vi "DAQ simulation.vi"(5 "Sampling rate":dbl=18000.0, 7 "Samples per channel":i32=500, 8 "Delay time (Pulse width) ms":i32=10, 9 "index (row)":i32, 11 "Input data":dbl[][](array[numeric])) -> (1 "Stop":bool, 3 "Output":dbl[](array[numeric]))   [LabVIEW 2018]
panel:
  out "Waveform Graph":dbl[](graph)
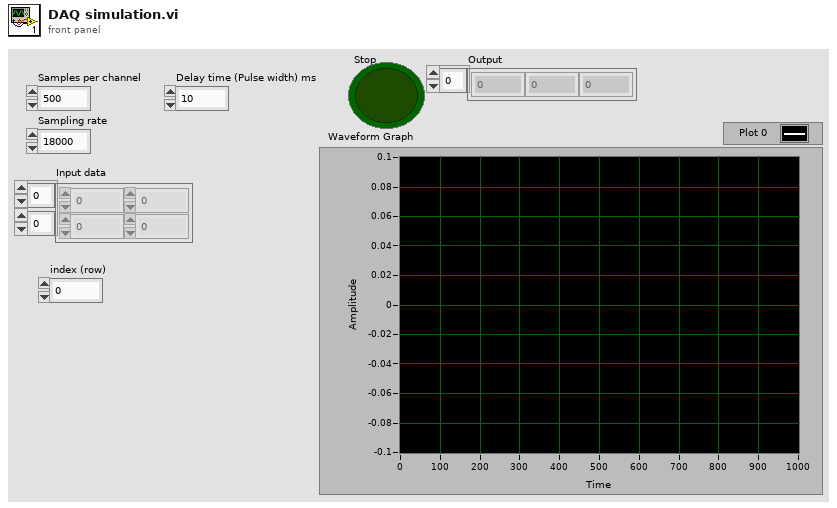
[diagram p1: front panel]
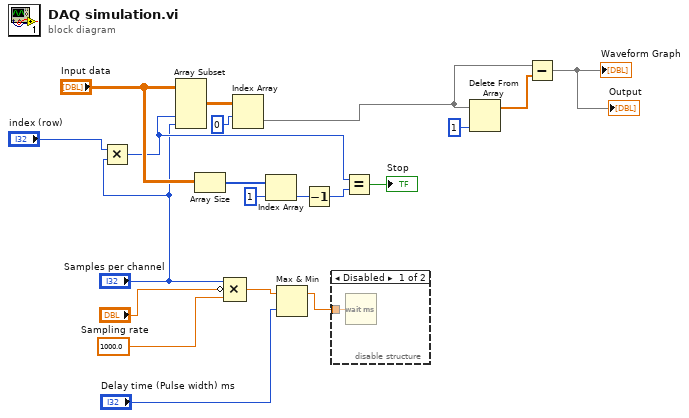
[diagram p0: block diagram]
diagram:
  n1 = Multiply(x="index (row)", y="Samples per channel") -> (x*y=w6:i32)
  n2 = Array Subset(array="Input data", index (col)=w6, length (col)="Samples per channel") -> (w9:dbl[][])  [unwired: 2 in]
  n3 = Array Size(array="Input data") -> (size(s)=w19:i32[])
  n4 = Compound Arithmetic op=MULTIPLY("Samples per channel", invert "Sampling rate", 1000.0 ("value")) -> (w12:dbl)
  n5 = Index Array(array=w9, index (row)=0 ("disabled index (col)")) -> (element=w3:dbl[])  [unwired: 1 in]
  n6 = Index Array(array=w19, index=1) -> (element=w18:i32)
  n7 = Max & Min(x=w12, y="Delay time (Pulse width) ms") -> (max(x,y)=w10:dbl)  [unwired: 1 out]
  n8 = Decrement(x=w18) -> (x-1=w17:i32)
  n9 = disable-structure shown="Disabled" {
    disable-tunnel: w10 -> [w21 _]
    frame Disabled {
      n10 = Wait (ms)(milliseconds to wait=w21) -> ()  [unwired: 1 out]
    }
    frame Enabled {
    }
  }
  n11 = Equal?(x=w6, y=w17) -> (x = y?=→"Stop":bool)
  n12 = Delete From Array(array=w3, index=1) -> (array with subset deleted=w2:dbl[])  [unwired: 1 in, 1 out]
  n13 = Subtract(x=w3, y=w2) -> (x-y=→"Output" →"Waveform Graph":dbl[])
